vi "sub_Generate_Packet_Array.vi"(0 "Packet Parameters":T1, 1 "PN sequence order\nfor Sync":i32=9 caption="PN sequence order (9)", 7 "Packet Number":i32, 9 "User defined bitstream?":bool=TRUE, 12 "user  bitstream":i8[](array[numeric])=[1], 14 "Cyclic Padding Bits":i32) -> (4 "Output Packet":i8[](array[numeric]))   [LabVIEW 2011]
uses:
  <vilib>/addons/Modulation/Digital/General/MT Generate Bits (Galois, PN Order).vi
  <vilib>/addons/Modulation/niDMT.lvlib
panel:
  out "error out":errorcluster
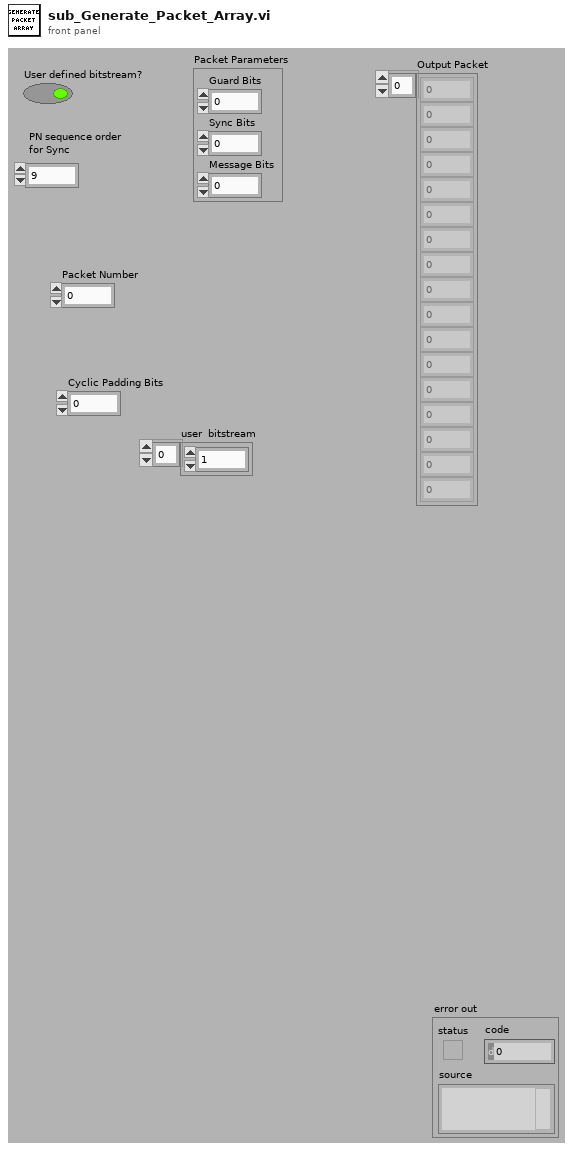
[diagram p1: front panel]
types:
  T1 = cluster{"Guard Bits ":i32, "Sync Bits":i32, "Message Bits":i32}
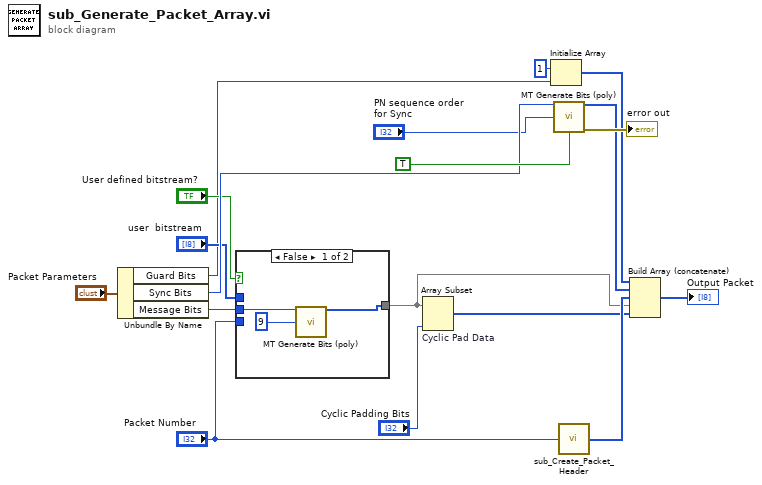
[diagram p0: block diagram]
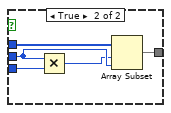
[diagram p2: hidden frame]
diagram:
  n1 = Unbundle By Name("Packet Parameters") -> ("Guard Bits"=w3:i32, "Sync Bits"=w15:i32, "Message Bits"=w13:i32)
  n2 = case shown="False" "User defined bitstream?" {
    tunnel: w13 -> [w20 w24]
    tunnel: [w19 w22] -> w5
    tunnel: "Packet Number" -> [_ w26]
    tunnel: "user  bitstream" -> [_ w25]
    frame False {
      n3 = call-poly <vilib>:"MT Generate Bits (poly).vi"("total bits (128)"=w20, "PN sequence order (9)"=9) -> ("output bit stream"=w19:i8[])  [unwired: 3 in, 10 out]
    }
    frame True {
      n4 = Multiply(x=w24, y=w26) -> (x*y=w23:i32)
      n5 = Array Subset(array=w25, index=w23, length=w24) -> (w22:i8[])
    }
  }
  n6 = Array Subset "Cyclic Pad Data"(array=w5, length="Cyclic Padding Bits") -> (w4:i8[])  [unwired: 1 in]
  n7 = Initialize Array(i8 1 ("Numeric"), w3) -> (w1:i8[])
  n8 = call-poly <vilib>:"MT Generate Bits (poly).vi"("total bits (128)"=w15, "PN sequence order (9)"="PN sequence order\nfor Sync", "reset? (T)"=TRUE ("Reset? (T)")) -> ("output bit stream"=w9:i8[], "error out"=→"error out":errorcluster)  [unwired: 10 in, 1 out]
  n9 = call "sub_Create_Packet_Header.vi"("Packet Number"="Packet Number") -> ("Array"=w14:i8[])
  n10 = Build Array (concatenate)(w1, w9, w14, w5, w4) -> (→"Output Packet":i8[])
